vi "Send2DGotoComm.vi"(6 "YParInstInd":i32, 8 "error in (no error)":errorcluster caption="entrée d'erreur (pas d'erreur)", 9 "XY Data":dbl[](array[numeric]), 10 "XParInstInd":i32, 11 "Interface en entrée":refnum<class "Interface.lvclass"> caption="DNL_LabVIEW Object in") -> (0 "error out":errorcluster caption="sortie d'erreur", 3 "Interface en sortie":refnum<class "Interface.lvclass"> caption="DNL_LabVIEW Object out")   [LabVIEW 2019, in "Interface.lvclass"]
uses:
  Interface.lvclass
  Interface.lvclass/Interface.ctl
  Experiment Class/Experiment.lvclass
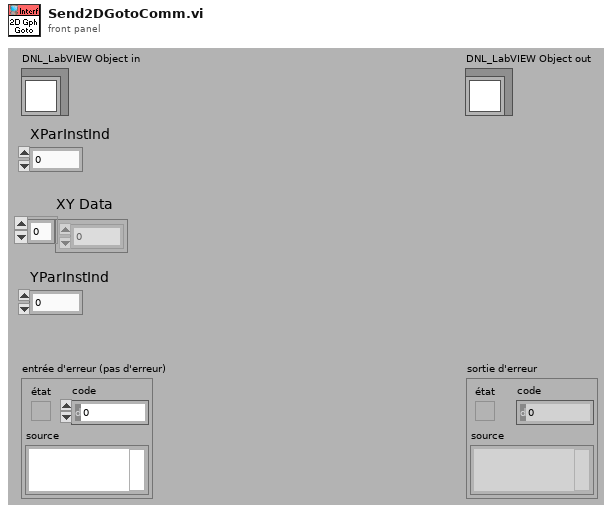
[diagram p1: front panel]
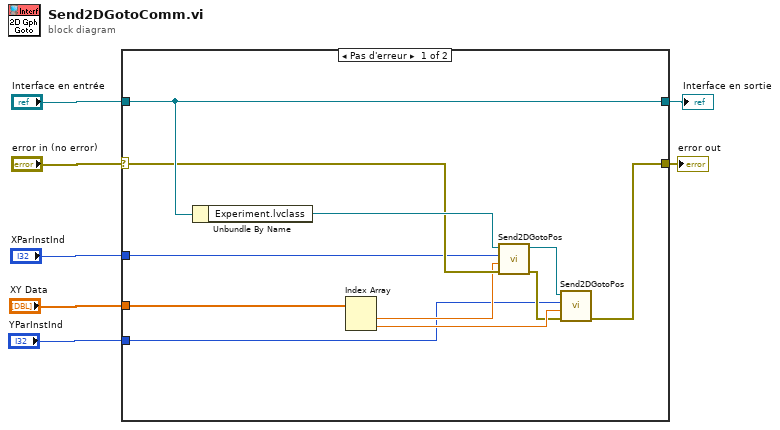
[diagram p0: block diagram]
diagram:
  n1 = case shown="Pas d'erreur" "error in (no error)" {
    selector: "error in (no error)" -> [w16 w20]
    tunnel: [w15 w20] -> w6
    tunnel: [w18 w19] -> w4
    tunnel: "Interface en entrée" -> [w18 w19]
    tunnel: "XParInstInd" -> [w8 _]
    tunnel: "XY Data" -> [w14 _]
    tunnel: "YParInstInd" -> [w9 _]
    frame No Error {
      n2 = Unbundle By Name(w18) -> ("Experiment.lvclass"=w17:refnum<class "Experiment.lvclass">)
      n3 = Index Array(array=w14) -> (element #1=w12:dbl, element #2=w11:dbl)  [unwired: 2 in]
      n4 = call "Send2DGotoPos.vi"("error in (no error)"=w16, "GotoPos"=w12, "InstrIndex"=w8, "Experiment en entrée"=w17) -> ("error out"=w10:errorcluster, "Experiment en sortie"=w13:refnum<class "Experiment.lvclass">)  [unwired: 6 in]
      n5 = call "Send2DGotoPos.vi"("error in (no error)"=w10, "GotoPos"=w11, "InstrIndex"=w9, "Experiment en entrée"=w13) -> ("error out"=w15:errorcluster)  [unwired: 6 in, 1 out]
    }
    frame Error {
    }
  }
  "error out" <- w6
  "Interface en sortie" <- w4
